vi "ChildImplementationINIKey--Constant.vi"() -> (3 "ChildImplementationPathKey":string)   [LabVIEW 2021, in "lv_icon.lvlib"]
uses:
  <vilib>/LabVIEW Icon API/lv_icon/lv_icon.lvlib
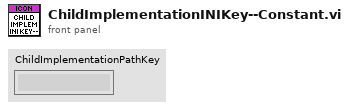
[diagram p1: front panel]
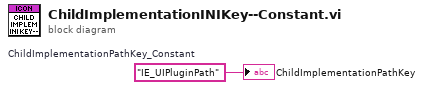
[diagram p0: block diagram]
diagram:
  w1 = "IE_UIPluginPath"  # ChildImplementationPathKey_Constant
  "ChildImplementationPathKey" <- w1
